vi "Start Sync.vi"(8 "error in (no error)":errorcluster, 11 "gRPC service in":refnum<class "ExamplePluginOOBService.lvclass">) -> (0 "error out":errorcluster, 3 "gRPC service out":refnum<class "ExamplePluginOOBService.lvclass">)   [LabVIEW 2025, in "Automotive-Vision-OOBService_server.lvlib" / "ExamplePluginOOBService.lvclass"]
uses:
  ExamplePluginOOBService.lvclass
  ExamplePluginOOBService.lvclass/ExamplePluginOOBService.ctl
  Automotive-Vision OOB Data Transfer/Automotive-Vision OOB Data Transfer.lvlib
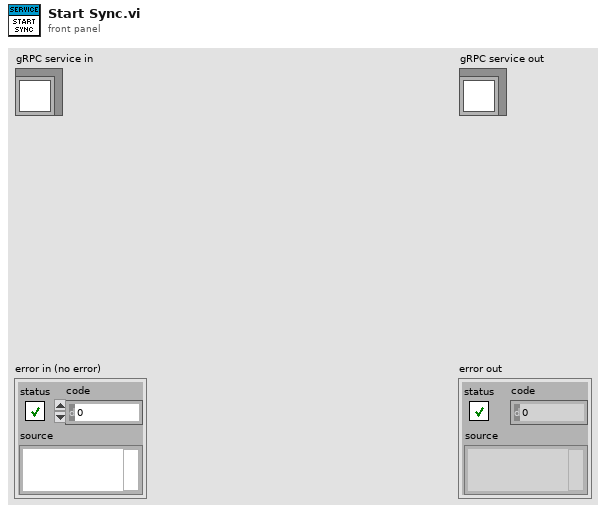
[diagram p1: front panel]
types:
  T1 = typedef "Automotive-Vision-OOBService_server.lvlib/ExamplePluginOOBService.lvclass/Server Internal UEs.ctl" = cluster{"ExamplePluginOOBService PauseResume Internal UE":refnum<user-event>, "ExamplePluginOOBService ExportPath Internal UE":refnum<user-event>, "ExamplePluginOOBService ExportType Internal UE":refnum<user-event>, "ExamplePluginOOBService Export Internal UE":refnum<user-event>}
  T2 = typedef "Automotive-Vision-OOBService_server.lvlib/ExamplePluginOOBService.lvclass/Server gRPC UEs.ctl" = cluster{"ExamplePluginOOBService PauseResume gRPC UE":refnum<user-event>, "ExamplePluginOOBService ExportPath gRPC UE":refnum<user-event>, "ExamplePluginOOBService ExportType gRPC UE":refnum<user-event>, "ExamplePluginOOBService Export gRPC UE":refnum<user-event>}
  T3 = typedef "grpc-lvsupport-release.lvlib/grpcId.ctl" = u64
  T4 = typedef "Automotive-Vision OOB Data Transfer.lvlib/OOB to Logic Data.ctl" = cluster{"PauseResume":bool, "ExportPath":string, "ExportType":u16, "Export":bool}
  T5 = typedef "Automotive-Vision-OOBService_server.lvlib/hwval_BoolRequest.ctl" = cluster{"BooleanData":bool}
  T6 = typedef "Automotive-Vision-OOBService_server.lvlib/hwval_ExportRequest.ctl" = cluster{"FilePath":string}
  T7 = typedef "Automotive-Vision-OOBService_server.lvlib/hwval_ExportTypeRequest.ctl" = cluster{"FileType":T8}
  T8 = typedef "Automotive-Vision-OOBService_server.lvlib/hwval_ExportFileType.ctl" = enum32{"EXPORT_PNG", "EXPORT_RAW"}
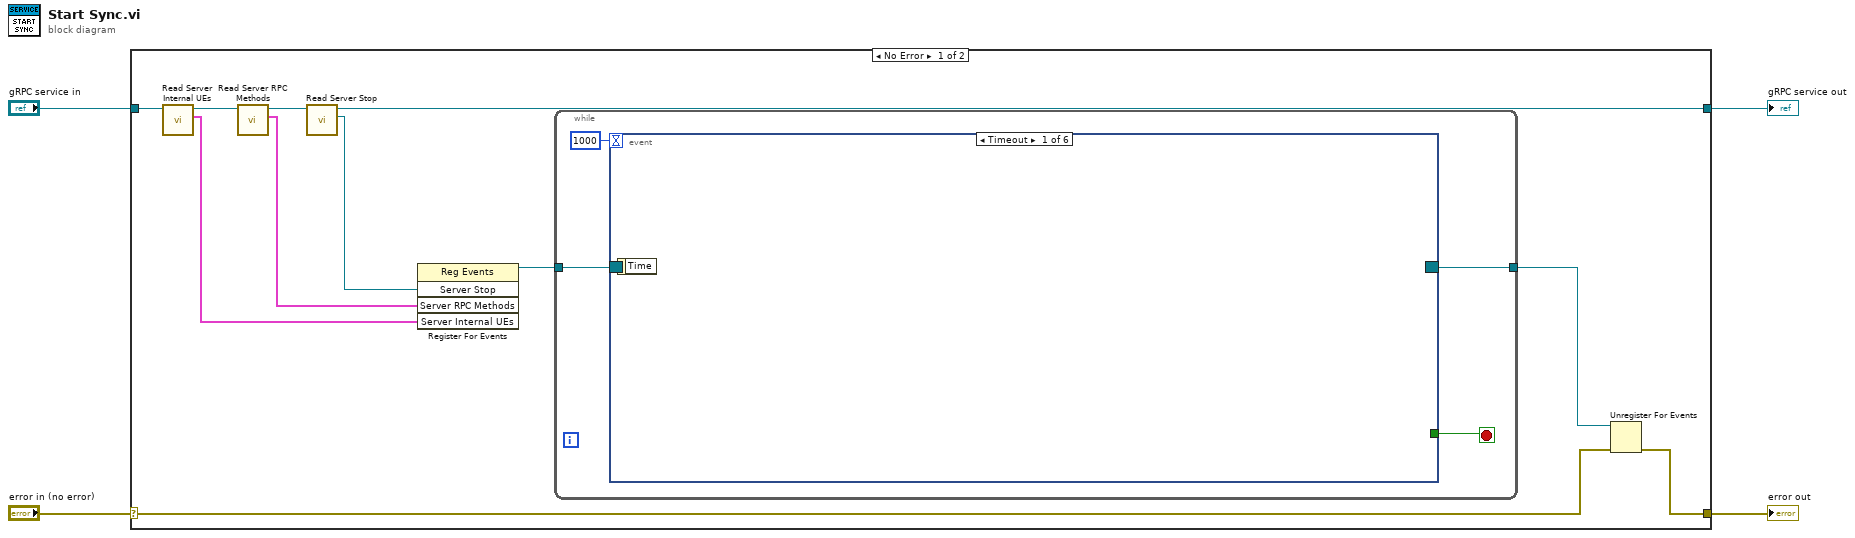
[diagram p0: block diagram]
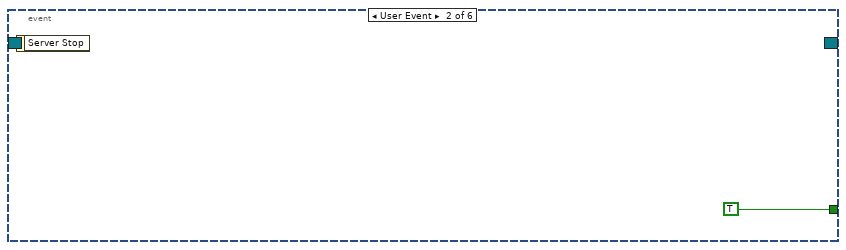
[diagram p2: hidden frame]
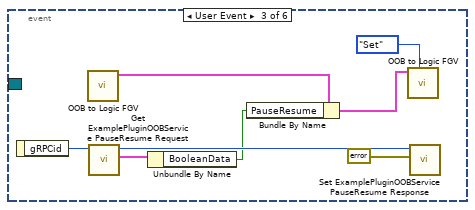
[diagram p3: hidden frame]
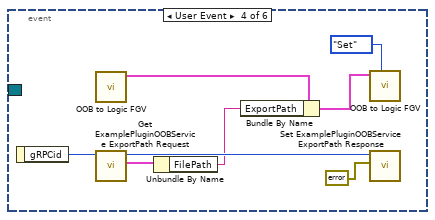
[diagram p4: hidden frame]
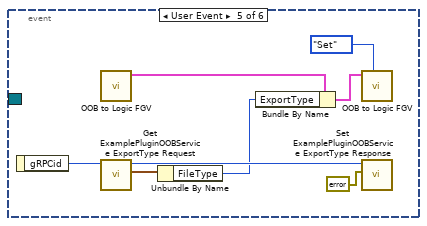
[diagram p5: hidden frame]
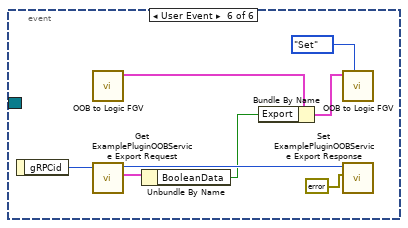
[diagram p6: hidden frame]
diagram:
  n1 = case shown="No Error" "error in (no error)" {
    selector: "error in (no error)" -> [w9 w54]
    tunnel: [w8 w54] -> w3
    tunnel: [w6 w53] -> w1
    tunnel: "gRPC service in" -> [w15 w53]
    frame No Error {
      n2 = call "Read Server Internal UEs.vi"("gRPC service in"=w15) -> ("Server Internal UEs"=w13:T1, "gRPC service out"=w14:refnum<class "ExamplePluginOOBService.lvclass">)  [unwired: 8 in, 1 out]
      n3 = call "Read Server RPC Methods.vi"("gRPC service in"=w14) -> ("Server RPC Methods"=w7:T2, "gRPC service out"=w12:refnum<class "ExamplePluginOOBService.lvclass">)  [unwired: 8 in, 1 out]
      n4 = call-dynamic "Read Server Stop.vi"("gRPC service in"=w12) -> ("Server Stop"=w5:refnum<user-event>, "gRPC service out"=w6:refnum<class "ExamplePluginOOBService.lvclass">)  [unwired: 8 in, 1 out]
      n5 = register-events(w5, w7, w13) -> (reference out=w11:refnum<event-registration>)  [unwired: 2 in, 1 out]
      n6 = while {
        tunnel: w11 -> [w19]
        tunnel: [w17] -> w10
        stop <- w18 stop-if-true
        n7 = event "RPC Methods Event Structure" shown="[0] Timeout" {
          selector: w19 -> [_ _ _ _ _ _]
          dyn-events: [_ _ _ _ _ _] -> w17
          timeout: 1000 -> [_ _ _ _ _ _]
          tunnel: [_ TRUE _ _ _ _] -> w18
          event Timeout {
            n8 = event-data() -> ()  [unwired: 1 in, 1 out]
          }
          event User Event {
            n9 = event-data() -> ()  [unwired: 1 in, 1 out]
          }
          event User Event {
            n10 = event-data() -> ("gRPCid"=w28:T3)  [unwired: 1 in]
            n11 = call "OOB to Logic FGV.vi"() -> ("OOB to Logic Data out"=w27:T4)  [unwired: 10 in, 1 out]
            n12 = call "Get ExamplePluginOOBService PauseResume Request.vi"("gRPCid"=w28) -> ("Message Data"=w22:T5, "gRPCid out"=w26:T3)  [unwired: 8 in, 1 out]
            n13 = Unbundle By Name(w22) -> ("BooleanData"=w21:bool)
            n14 = Bundle By Name(cluster=w27, "PauseResume"=w21) -> (w24:T4)
            n15 = call "OOB to Logic FGV.vi"("Op (Get)"=enum16{"Get", "Set"}."Set", "OOB to Logic Data in"=w24) -> ()  [unwired: 8 in, 2 out]
            n16 = call "Set ExamplePluginOOBService PauseResume Response.vi"("Message Data"=errorcluster {"status"=FALSE, "code"=0, "source"=""} ("error in (no error)"), "gRPCid in"=w26) -> ()  [unwired: 9 in, 1 out]
          }
          event User Event {
            n17 = event-data() -> ("gRPCid"=w36:T3)  [unwired: 1 in]
            n18 = call "OOB to Logic FGV.vi"() -> ("OOB to Logic Data out"=w33:T4)  [unwired: 10 in, 1 out]
            n19 = call "Get ExamplePluginOOBService ExportPath Request.vi"("gRPCid"=w36) -> ("Message Data"=w34:T6, "gRPCid out"=w35:T3)  [unwired: 8 in, 1 out]
            n20 = Unbundle By Name(w34) -> ("FilePath"=w32:string)
            n21 = Bundle By Name(cluster=w33, "ExportPath"=w32) -> (w31:T4)
            n22 = call "OOB to Logic FGV.vi"("Op (Get)"=enum16{"Get", "Set"}."Set", "OOB to Logic Data in"=w31) -> ()  [unwired: 8 in, 2 out]
            n23 = call "Set ExamplePluginOOBService ExportPath Response.vi"("Message Data"=errorcluster {"status"=FALSE, "code"=0, "source"=""} ("error in (no error)"), "gRPCid in"=w35) -> ()  [unwired: 9 in, 1 out]
          }
          event User Event {
            n24 = event-data() -> ("gRPCid"=w44:T3)  [unwired: 1 in]
            n25 = call "OOB to Logic FGV.vi"() -> ("OOB to Logic Data out"=w41:T4)  [unwired: 10 in, 1 out]
            n26 = call "Get ExamplePluginOOBService ExportType Request.vi"("gRPCid"=w44) -> ("Message Data"=w42:T7, "gRPCid out"=w43:T3)  [unwired: 8 in, 1 out]
            n27 = Unbundle By Name(w42) -> ("FileType"=w40:T8)
            n28 = Bundle By Name(cluster=w41, "ExportType"=w40) -> (w39:T4)
            n29 = call "OOB to Logic FGV.vi"("Op (Get)"=enum16{"Get", "Set"}."Set", "OOB to Logic Data in"=w39) -> ()  [unwired: 8 in, 2 out]
            n30 = call "Set ExamplePluginOOBService ExportType Response.vi"("Message Data"=errorcluster {"status"=FALSE, "code"=0, "source"=""} ("error in (no error)"), "gRPCid in"=w43) -> ()  [unwired: 9 in, 1 out]
          }
          event User Event {
            n31 = event-data() -> ("gRPCid"=w52:T3)  [unwired: 1 in]
            n32 = call "OOB to Logic FGV.vi"() -> ("OOB to Logic Data out"=w50:T4)  [unwired: 10 in, 1 out]
            n33 = call "Get ExamplePluginOOBService Export Request.vi"("gRPCid"=w52) -> ("Message Data"=w49:T5, "gRPCid out"=w51:T3)  [unwired: 8 in, 1 out]
            n34 = Unbundle By Name(w49) -> ("BooleanData"=w48:bool)
            n35 = Bundle By Name(cluster=w50, "Export"=w48) -> (w47:T4)
            n36 = call "OOB to Logic FGV.vi"("Op (Get)"=enum16{"Get", "Set"}."Set", "OOB to Logic Data in"=w47) -> ()  [unwired: 8 in, 2 out]
            n37 = call "Set ExamplePluginOOBService Export Response.vi"("Message Data"=errorcluster {"status"=FALSE, "code"=0, "source"=""} ("error in (no error)"), "gRPCid in"=w51) -> ()  [unwired: 9 in, 1 out]
          }
        }
      }
      n38 = Unregister For Events(event registration refnum=w10, error in=w9) -> (error out=w8:errorcluster)
    }
    frame Error {
    }
  }
  "error out" <- w3
  "gRPC service out" <- w1
